vi "Dashboard Main.vi"() -> ()   [LabVIEW 2015]
uses:
  Camera Types.ctl
  <vilib>/Utility/miscctls.llb/LVRowAndColumnTypeDef.ctl
  <vilib>/event_ctls.llb/eventvkey.ctl
  <vilib>/Rock Robotics/WPI/Dashboard/WPI_DashboardLogging Global.vi
  <vilib>/Rock Robotics/Network Tables/NT Read Boolean.vi
  <vilib>/Utility/file.llb/Write Delimited Spreadsheet (DBL).vi
  <vilib>/Rock Robotics/Network Tables/NT Write Numeric Array.vi
  <vilib>/Utility/file.llb/Read Delimited Spreadsheet (DBL).vi
  <vilib>/Rock Robotics/Network Tables/NT Write Boolean.vi
  <vilib>/Utility/config.llb/Write Key (String).vi
  <vilib>/Utility/config.llb/Write Key (I32).vi
  <vilib>/Utility/config.llb/NI_LVConfig.lvlib
  <vilib>/vision/NI_Vision_Development_Module.lvlib
panel:
  in  "Dashboard Tab":T1(tab)=enum."Commands"
  in  "Left / Right":bool
  out "Compass":dbl(knob) scale=-180.0..180.0
  out "Aimed?":bool
  out "position":dbl
  out "defense":dbl
  out "Have ball?":bool
  in  "Camera Settings":T2={"Frame Rate"=30, "Compression"=30, "Size"=1} {"Frame Rate" scale=1.0..30.0; "Size" items=["640x480", "320x240", "160x120"]}
  out "Mode":T3(ring)=enum."Auto Disabled"
  in  "DB Camera Config":bool
  out "fps":dbl format="%#.1g"
  out "Mbps":dbl format="%#.1g"
  out "Mbps LED":bool
  in  "Auto Position":i32(slide)=1 scale=1.0..5.0
  in  "Auto Defense":T4(ring)=enum."Low Bar"
  out "Detected Targets":T5(array[cluster]) {"Normalized Rect"."Numeric 5" format="%#_2g"; "Normalized Rect"."Numeric 3" format="%#_2g"; "Normalized Rect"."Numeric 2" format="%#_2g"; "Normalized Rect"."Numeric" format="%#_2g"}
  out "Masked":T6(plugin-control)
  out "Background":bool
  out "Qualified Particles":i32
  out "Highest Avg Score":dbl format="%#_3g"
  in  "Std Devs for Calibration":cluster{"H":dbl, "S":dbl, "V":dbl}={"H"=4.0, "S"=6.0, "V"=6.0}
  in  "Rec Mode":enum32{"Stop", "Record", "Playback"}(radio)
  in  "camSwitch?":bool
  in  "LED Color":T7={"Hue"={110.52399131877658, 148.6727294921875}, "Sat"={34.78571428571429, 255.0}, "Val"={91.07142857142858, 255.0}} {"Hue" scale=0.0..255.0 scale format="%_1f"}
  in  "Annotate":bool=TRUE
  in  "Annotation Limit":dbl=75.0
  in  "Aspect Ratio Fudge Factor":dbl=1.0
  in  "Min Score Threshold":i32=70
  in  "Camera Type":T8=enum."1013"
  in  "Emphasize Limit Tests":bool=TRUE
  in  "Green BCG Values":T9={"Brightness"=128.0, "Contrast"=45.0, "Gamma"=1.0} {"Brightness" min=0 max=255 step=1 format="%.2f"; "Contrast" min=1 max=89 step=1 format="%.2f"; "Gamma" min=0.1 max=10 step=0.01 format="%.2f"}
  in  "Blue BCG Values":T9={"Brightness"=128.0, "Contrast"=45.0, "Gamma"=1.0} {"Brightness" min=0 max=255 step=1 format="%.2f"; "Contrast" min=1 max=89 step=1 format="%.2f"; "Gamma" min=0.1 max=10 step=0.01 format="%.2f"}
  in  "Red BCG Values":T9={"Brightness"=128.0, "Contrast"=45.0, "Gamma"=1.0} {"Brightness" min=0 max=255 step=1 format="%.2f"; "Contrast" min=1 max=89 step=1 format="%.2f"; "Gamma" min=0.1 max=10 step=0.01 format="%.2f"}
  in  "Vision":u16(ring) items=["Camera Off", "USB Camera SW", "USB Camera HW", "IP Camera"]
  in  "Save?":bool
  out "Tree":string(tree)
  in  "Test Slider":dbl(slide) scale=0.0..100.0 scale format="%#_3g"
  in  "On/Off":bool caption="Solenoid"
  in  "Test Name":u16(ring) items=["Select the test to run..."]
  in  "Test Tree":string(tree)
  in  "Motor":cluster{"Value":dbl, "Enable":bool} {"Value" scale=-1.0..1.0 scale format="%#_3g"}
  out "Progress":T10 {"Test Progress" scale=0.0..100.0}
  in  "Rev/Fwd":cluster{"Forward":bool, "Reverse":bool}
  in  "Test Ring":u16(ring) items=["Monochrome", "Color"]
  out "Cmd Status":string
  in  "Execute Command":bool
  in  "Command Params":string[][](table)
  in  "Command Selection":i32(listbox)
  out "NT Connection":bool
  in  "Select Auto":string(combo)
  in  "CheckList":i32(listbox)
  out "Original Image":T6(plugin-control)
  out "Camera Image":T6(plugin-control)
  in  "TCP":refnum<k5>
  out "Camera IP":string
  out "Image Message":string="Timeout in Camera Communications"
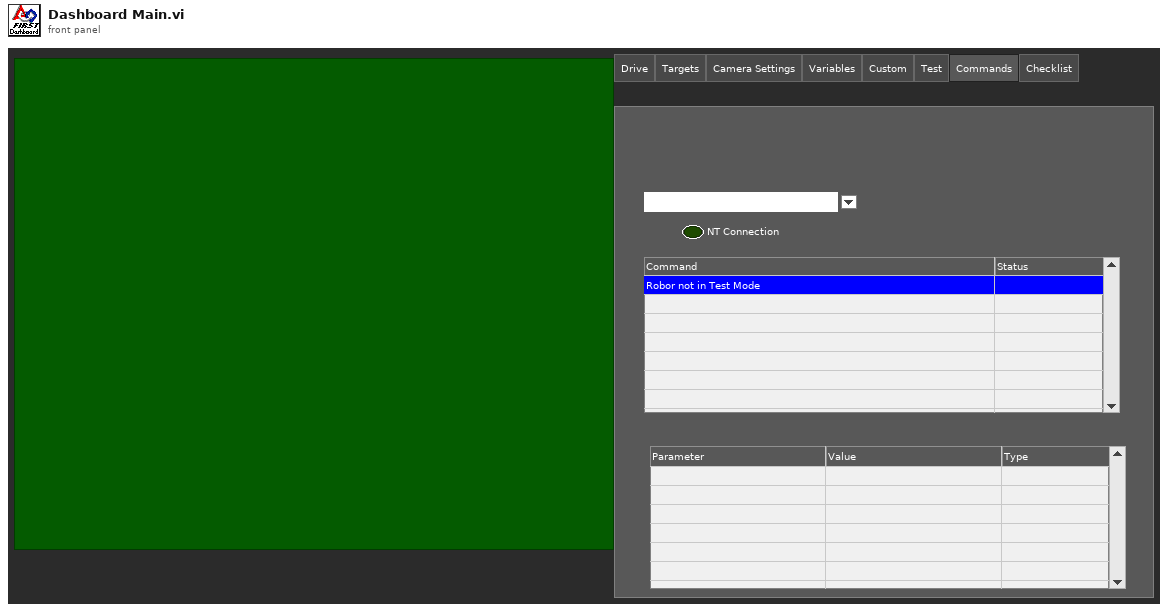
[diagram p1: front panel]
types:
  T1 = enum32{"Drive", "Targets", "Camera Settings", "Variables", "Custom", "Test", "Commands", "Checklist"}
  T2 = cluster{"Frame Rate":i32, "Compression":i32, "Size":u16}
  T3 = enum8{"Tele-Op Disabled", "Tele-Op Enabled", "Auto Disabled", "Auto Enabled", "Test Disabled", "Test Enabled", "Disconnected", "No Code", "E-Stop"}
  T4 = enum16{"Portcullis", "Cheval de Frise", "Low Bar", "Rock Wall", "Rough Terrain", "Moat", "Ramparts", "Vision Low Bar", "2-ball", "Do Nothing"}
  T5 = cluster{"Distance (ft)":dbl, "Center":cluster{dbl, dbl}, "Normalized Rect":cluster{"Numeric":dbl, "Numeric 2":dbl, "Numeric 3":dbl, "Numeric 5":dbl}}[]
  T6 = typedef "IMAQ Image.ctl" = refnum<image>
  T7 = cluster{"Hue":cluster{dbl, dbl}, "Sat":cluster{dbl, dbl}, "Val":cluster{dbl, dbl}}
  T8 = typedef "Camera Types.ctl" = enum16{"206", "1011", "1013", "MS HD3000 square", "MS HD3000 640x480"}
  T9 = cluster{"Brightness":sgl, "Contrast":sgl, "Gamma":sgl}
  T10 = cluster{"Test Progress":u8, "Test Progress Text":string}
  T11 = typedef "Image Type" = u32
  T12 = cluster{"IDs":cluster{"RPC field ID":u16, "Unique ID":u16}, "String":string}
  T13 = enum32{"Drive", "Basic", "Custom", "Test", "Checklist", "Variables"}
  T14 = cluster{cluster{"Numeric":dbl, "Numeric":dbl}, cluster{"Numeric":dbl, "Numeric":dbl}, cluster{"Numeric":dbl, "Numeric":dbl}}
  T15 = cluster{"Camera Image":refnum<vi>, "Dashboard Tab":refnum<vi>, "Background":refnum<vi>, "Vision":refnum<vi>, "Rec Mode":refnum<vi>, "Test Slider":refnum<vi>, "On/Off ":refnum<vi>, "Test Ring":refnum<vi>, "Rev/Fwd":refnum<vi>, "Test Name":refnum<vi>, "Motor":refnum<vi>, "Progress":refnum<vi>, "CheckList":refnum<vi>, "Tree":refnum<vi>, "Test Tree":refnum<vi>, "Command Params":refnum<vi>, "Command Selection":refnum<vi>, "Execute Command":refnum<vi>, "Cmd Status":refnum<vi>}
  T16 = typedef "Particle Parameters" = i32
  T17 = cluster{cluster{dbl, dbl}, cluster{dbl, dbl}, cluster{dbl, dbl}}
  T18 = cluster{"Bounding box":cluster{"left":dbl, "top":dbl, "right":dbl, "bottom":dbl}, "Aspect Ratio":dbl, "Area to CH":dbl, "X Mask":dbl, "Y Mask":dbl, "Moment":dbl}[]
  T19 = cluster{"Distance (ft)":dbl, "Center":cluster{dbl, dbl}, "Normalized Rect":cluster{"Numeric":dbl, "Numeric 2":dbl, "Numeric 3":dbl, "Numeric 5":dbl}}
  T20 = cluster{"Numeric":dbl, "Numeric 2":dbl, "Numeric 3":dbl, "Numeric 5":dbl}
  T21 = typedef "NI_LVConfig.lvlib/Config Data RefNum.ctl" = refnum<k1>
  T22 = cluster{"Error Strings":string, "Disable Counts":cluster{u16, u16}, "Rail Faults":cluster{u16, u16, u16}, "Robot IP":string, "DB Mode":u8, "Event Info":cluster{"Name":string, "Type":u8, "Number":u16, "Replay":u8}, "Camera Addr":string}
  T23 = cluster{"Storage":cluster{"Disk Free":u64, "RAM Block":u32, "RAM free":u32}, "CPU Utilization":cluster{"CPU % ISR":sgl, "CPU % Time Crit":sgl, "CPU % Timed Str":sgl, "CPU % High":sgl, "CPU % Above":sgl, "CPU % Normal":sgl, "CPU % Low":sgl}, "CAN":cluster{"% Bus Utilization":sgl, "Bus Off Cnt":u32, "TX_FIFO Full Cnt":u32, "Receive Error Cnt":u8, "Transmit Error Cnt":u8}, "HID":cluster{"HID Outputs":u32, "Rumble Low":u16, "Rumble High":u16}[]}
  T24 = cluster{"Status bits":cluster{"Test Mode":bool, "Autonomous":bool, "Enabled":bool, "Code Start":bool, "Brownout":bool, "Reserved 2":bool, "Reserved 3":bool, "E-Stop":bool}, "Code Trace":cluster{"Disabled":bool, "TeleOp":bool, "Auto":bool, "Test":bool}, "Controller Type":enum16{"unknown", "cRIO", "roboRio"}, "Code?":enum16{"unknown", "noCode", "code"}, "Battery V":dbl}
  T25 = cluster{"Control Bits":cluster{"TestMode":bool, "Autonomous":bool, "Enabled":bool, "FMS Present":bool, bool, bool, bool, "E-Stop":bool}, "Team Station ":u8, "Countdown":sgl, "Joystick Values":cluster{"Axes":dbl[], "Buttons":bool[], "POVs":i16[]}[]}
  T26 = cluster{"Operation":enum16{"Update", "Clear"}, "Color Box":u32}[]
  T27 = typedef "eventvkey.ctl" = enum16{"ASCII", "Enter", "Return", "Shift", "Ctrl", "Alt", "Cmd", "Opt", "Caps", "NumLock", "Clear", "Break", "Up", "Down", "Left", "Right", "Insert", "Delete", "Home", "End", "PageUp", "PageDown", "Escape", "Help", "Pause", "ScrollLock", "F1", "F2", "F3", "F4", "F5", "F6", "F7", "F8", "F9", "F10", "F11", "F12", "F13", "F14", "F15", "F16", "F17", "F18", "F19", "F20", "F21", "F22", "F23", "F24", "Play", "VolumeUp", "VolumeDown", "Mute", "Two Byte Char"}
  T28 = cluster{"Image Size":bool, "Image Type":bool, "Pixel Value":bool, "ROI Information":bool, "Zoom Factor":bool}
  T29 = enum8{"Enabled", "Disabled", "Disabled and Grayed Out"}
  T30 = cluster{"Operation":enum16{"Update", "Clear"}, "Color Box":u32}
  T31 = typedef "LVRowAndColumnTypeDef.ctl" = cluster{"Row":i32, "Column":i32}
  T32 = cluster{"Shift":bool, "Ctrl":bool, "Alt":bool, "Cmd":bool, "Opt":bool}
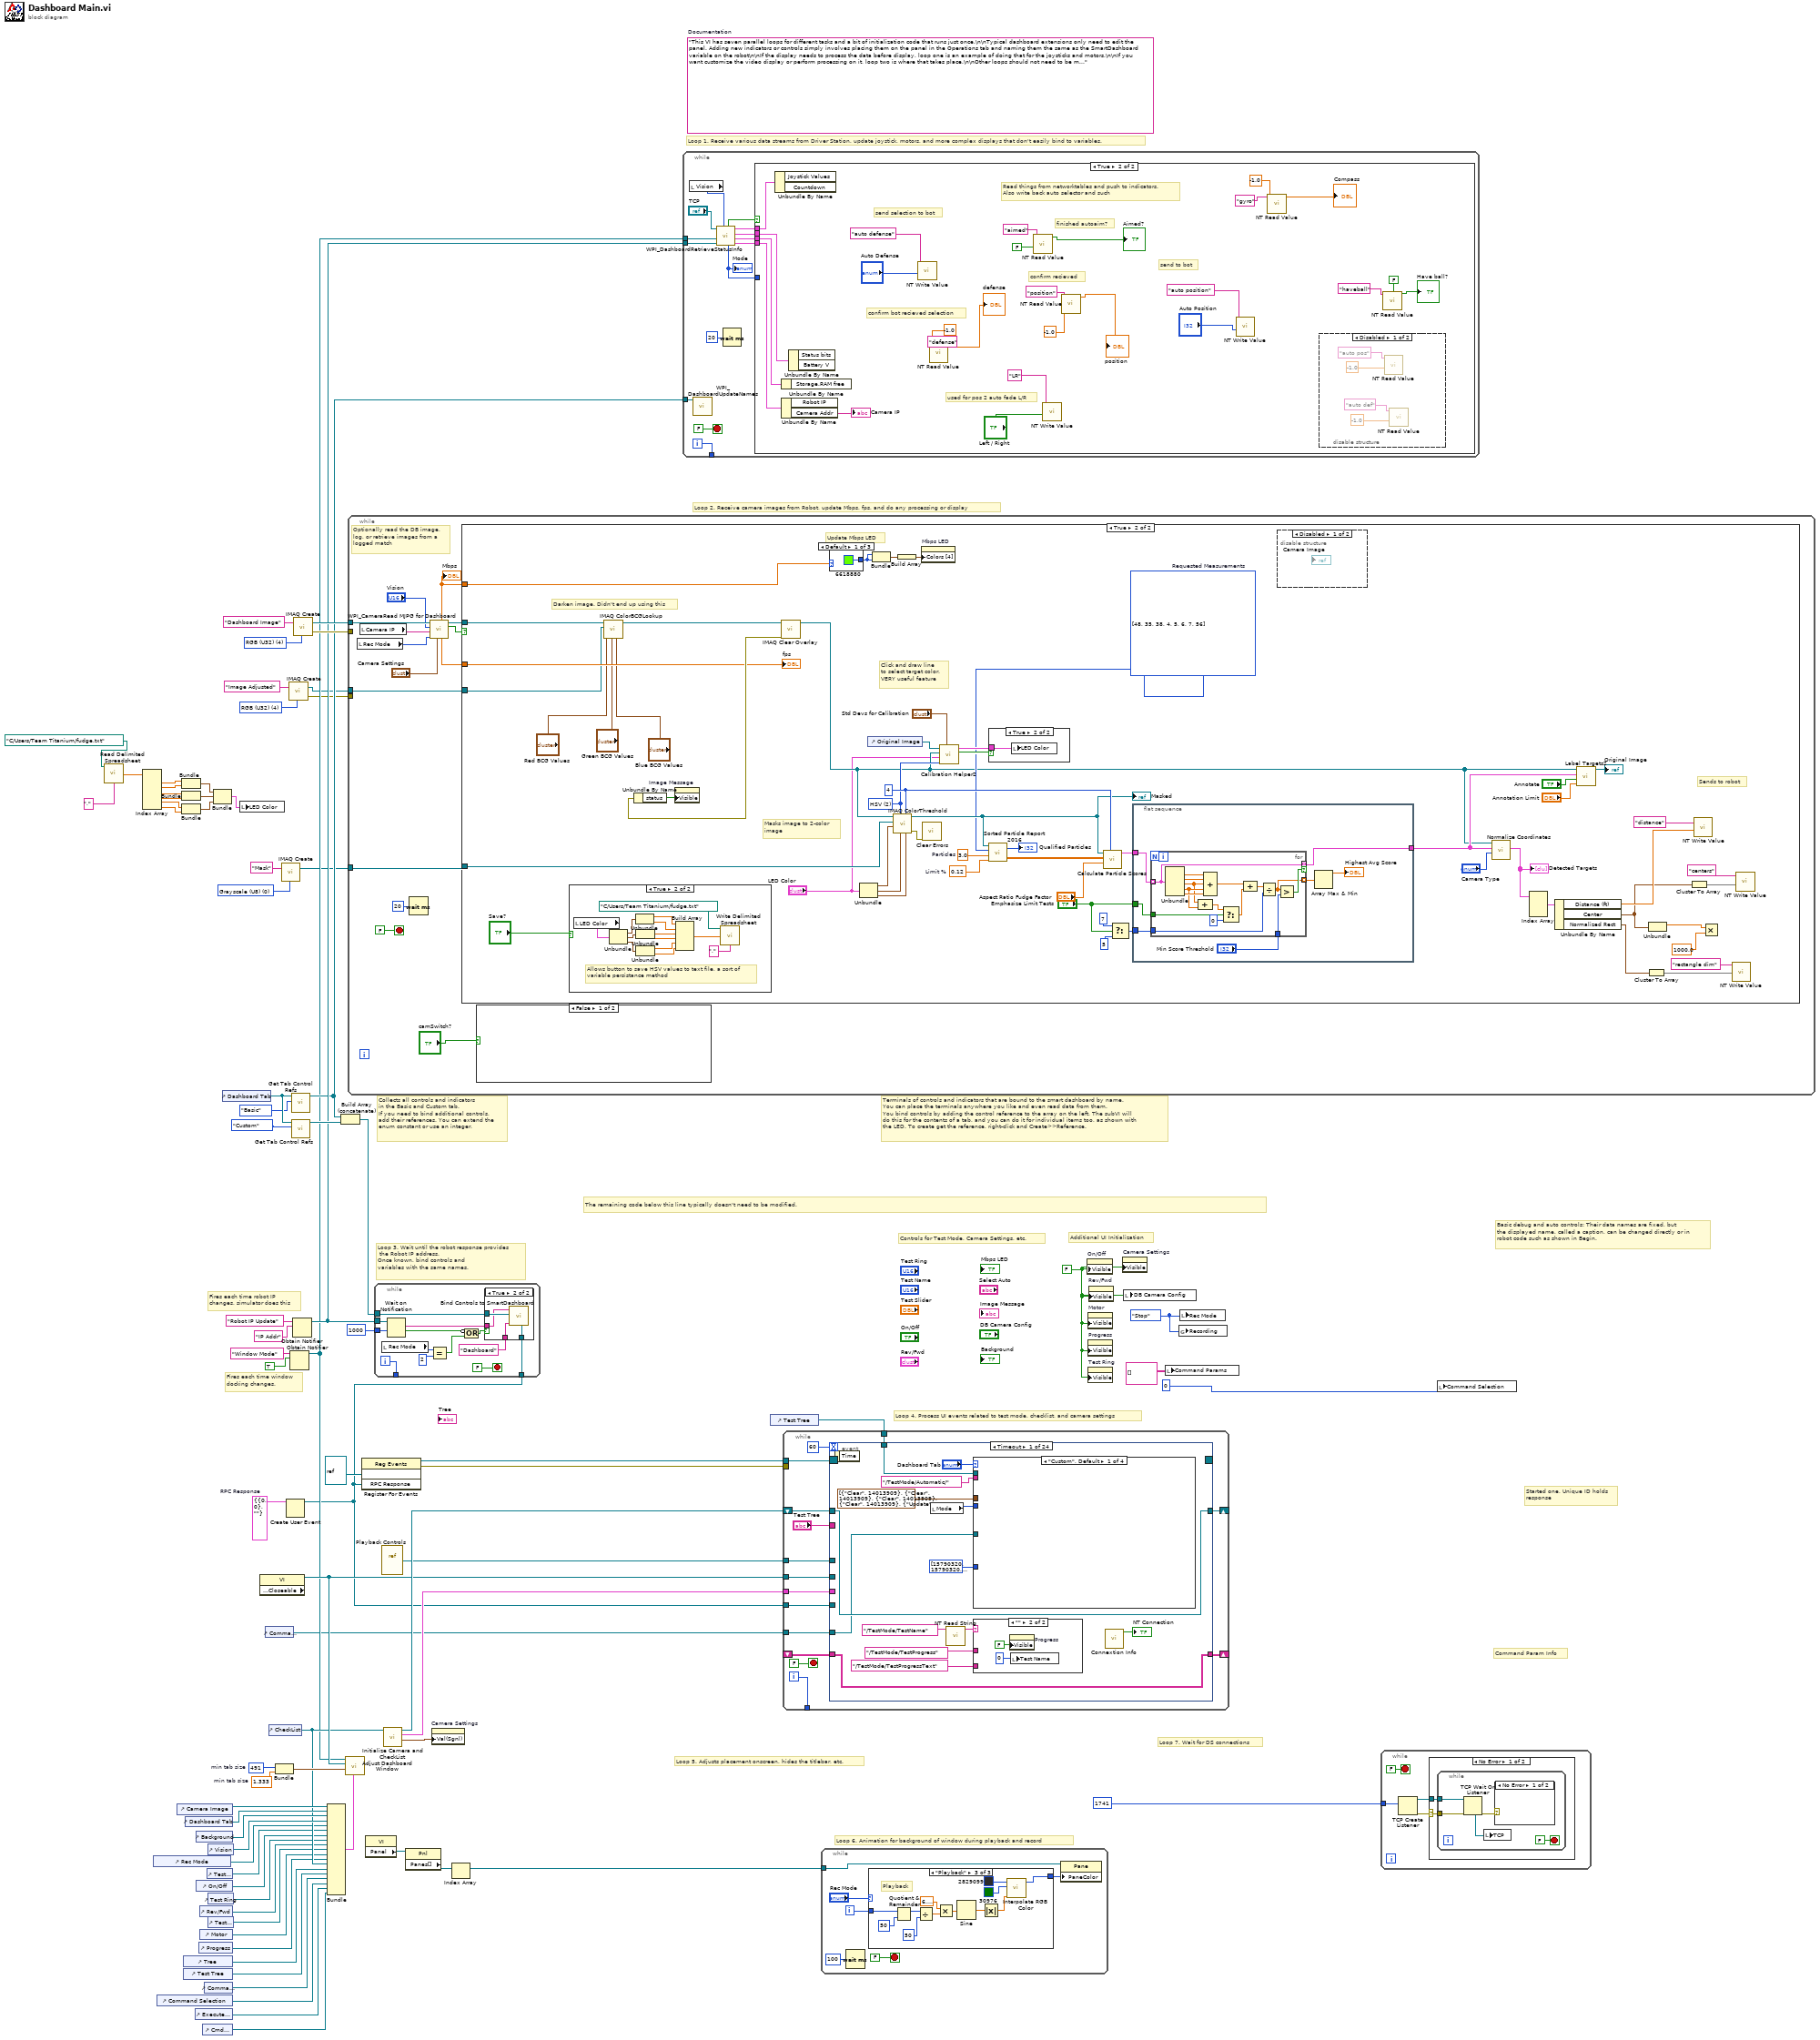
[diagram p0: block diagram]
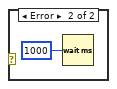
[diagram p2: hidden frame]
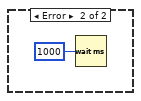
[diagram p3: hidden frame]
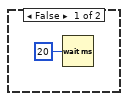
[diagram p4: hidden frame]
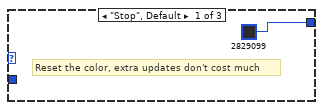
[diagram p6: hidden frame]
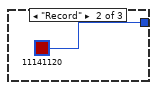
[diagram p7: hidden frame]
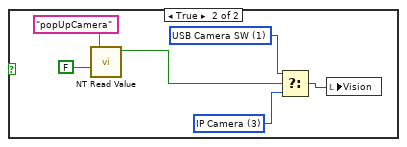
[diagram p9: hidden frame]
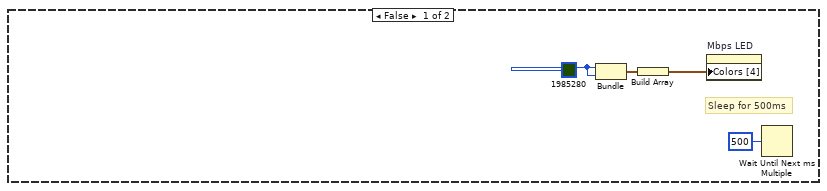
[diagram p10: hidden frame]
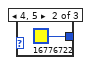
[diagram p14: hidden frame]
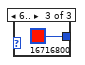
[diagram p15: hidden frame]
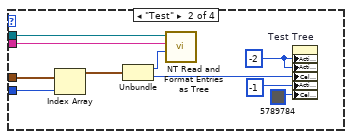
[diagram p16: hidden frame]
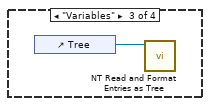
[diagram p17: hidden frame]
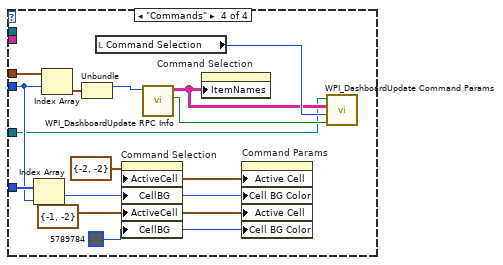
[diagram p18: hidden frame]
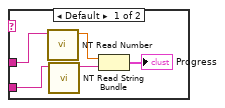
[diagram p19: hidden frame]
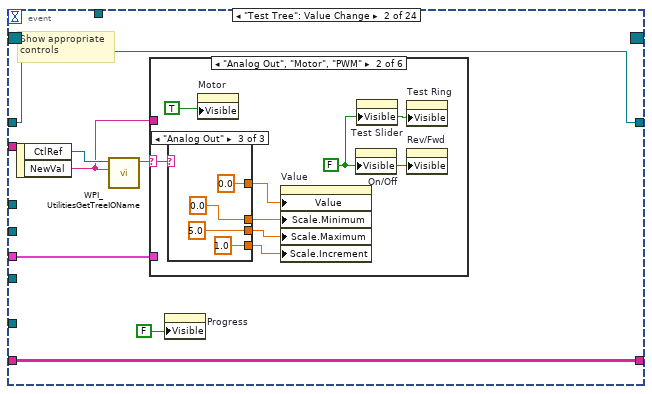
[diagram p20: hidden frame]
diagram:
  w17 = T11 4 items=["Grayscale (U8)", "Grayscale (I16)", "Grayscale (SGL)", "Complex (CSG)", "RGB (U32)", "HSL (U32)", "RGB (U64)"] ("Image Type")
  w19 = T11 0 items=["Grayscale (U8)", "Grayscale (I16)", "Grayscale (SGL)", "Complex (CSG)", "RGB (U32)", "HSL (U32)", "RGB (U64)", "Grayscale (U16)"] ("Image Type")
  w27 = T12 {"IDs"={"RPC field ID"=0, "Unique ID"=0}, "String"=""}  # RPC Response
  w52 = 491  # min tab size
  w51 = 1.333  # min tab size
  w60 = enum32{"Stop", "Record", "Playback"}."Stop" ("Rec Mode")
  w34 = FALSE ("Visible")
  (unwired) "This VI has seven parallel loops for different tasks and a bit of initialization code that runs just once.\n\nTypical dashboard extensions only need to edit the panel. Adding new indicators or controls simply involves placing them on the panel in the Operations tab and naming them the same as the SmartDashboard variable on the robot\n\nIf the display needs to process the data before display, loop one is an example of doing that for the joysticks and motors.\n\nIf you want customize the video display or perform processing on it, loop two is where that takes place.\n\nOther loops should not need to be modified. They are pretty standard, and document the task they perform."  # Documentation
  w80 = T11 4 items=["Grayscale (U8)", "Grayscale (I16)", "Grayscale (SGL)", "Complex (CSG)", "RGB (U32)", "HSL (U32)", "RGB (U64)"] ("Image Type")
  # "Command Param Info"
  # "Started one, Unique ID holds\nresponse"
  # "Loop 7. Wait for DS connections"
  # "Basic debug and auto controls: Their data names are fixed, but\nthe displayed name, called a caption, can be changed directly or in\nrobot code such as shown in Begin."
  # "Controls for Test Mode, Camera Settings, etc."
  # "Additional UI Initialization"
  # "Loop 6. Animation for background of window during playback and record"
  # "Fires each time robot IP\nchanges, simulator does this"
  # "Fires each time window\ndocking changes."
  # "Collects all controls and indicators\nin the Basic and Custom tab.\nIf you need to bind additional controls,\nadd their references. You can extend the\nenum constant or use an integer."
  # "The remaining code below this line typically doesn't need to be modified."
  # "Loop 4. Process UI events related to test mode, checklist, and camera settings"
  # "Terminals of controls and indicators that are bound to the smart dashboard by name.\nYou can place the terminals anywhere you like and even read data from them.\nYou bind controls by adding the control reference to the array on the left. The subVI will\ndo this for the contents of a tab, and you can do it for individual items too, as shown with\nthe LED. To create get the reference, right-click and Create>>Reference."
  # "Loop 3. Wait until the robot response provides\n the Robot IP address.\nOnce known, bind controls and\nvariables with the same names."
  # "Loop 5. Adjusts placement onscreen, hides the titlebar, etc."
  # "Loop 1. Receive various data streams from Driver Station, update joystick, motors, and more complex displays that don't easily bind to variables."
  # "Loop 2. Receive camera images from Robot, update Mbps, fps, and do any processing or display"
  n1 = call-poly <vilib>:"Read Delimited Spreadsheet.vi"("file path (dialog if empty)"=path "C:/Users/Team Titanium/fudge.txt", "delimiter (\\t)"="," ("delimiter (\\t)")) -> ("first row"=w12:dbl[])  [unwired: 8 in, 5 out]
  n2 = Index Array(array=w12) -> (element #1=w11:dbl, element #2=w10:dbl, element #3=w9:dbl, element #4=w8:dbl, element #5=w7:dbl, element #6=w6:dbl)  [unwired: 6 in]
  n3 = control-ref of="Rec Mode"() -> (w40:refnum<vi>)
  n4 = control-ref of="Command Selection"() -> (w26:refnum<vi>)
  n5 = control-ref of="Camera Image"() -> (w55:refnum<vi>)
  n6 = Bundle("Numeric"=w11, "Numeric"=w10) -> (w5:cluster{"Numeric":dbl, "Numeric":dbl})  [unwired: 1 in]
  n7 = Bundle("Numeric"=w9, "Numeric"=w8) -> (w4:cluster{"Numeric":dbl, "Numeric":dbl})  [unwired: 1 in]
  n8 = Bundle("Numeric"=w7, "Numeric"=w6) -> (w3:cluster{"Numeric":dbl, "Numeric":dbl})  [unwired: 1 in]
  n9 = control-ref of="Tree"() -> (w44:refnum<vi>)
  n10 = control-ref of="Test Tree"() -> (w43:refnum<vi>)
  n11 = control-ref of="Dashboard Tab"() -> (w54:refnum<vi>)
  n12 = control-ref of="Execute Command"() -> (w28:refnum<vi>)
  n13 = control-ref of="Background"() -> (w49:refnum<vi>)
  n14 = control-ref of="On/Off"() -> (w38:refnum<vi>)
  n15 = control-ref of="Progress"() -> (w35:refnum<vi>)
  n16 = control-ref of="Rev/Fwd"() -> (w36:refnum<vi>)
  n17 = control-ref of="Motor"() -> (w41:refnum<vi>)
  n18 = control-ref of="Cmd Status"() -> (w22:refnum<vi>)
  n19 = control-ref of="Command Params"() -> (w29:refnum<vi>)
  n20 = control-ref of="Test Slider"() -> (w39:refnum<vi>)
  n21 = control-ref of="Vision"() -> (w53:refnum<vi>)
  n22 = control-ref of="Test Ring"() -> (w37:refnum<vi>)
  n23 = control-ref of="Test Name"() -> (w42:refnum<vi>)
  n24 = Bundle(w5, w4, w3) -> (w2:T14)  [unwired: 1 in]
  n25 = control-ref of="Dashboard Tab"() -> (w58:refnum<vi>)
  n26 = local write "LED Color"(w2) -> ()
  n27 = property class="VI" props=["Front Panel.Closeable"]() -> (reference out=w59:refnum<vi>)  [unwired: 2 in, 2 out]
  n28 = control-ref of="Command Params"() -> (w21:refnum<vi>)
  n29 = control-ref of="CheckList"() -> (w45:refnum<vi>)
  n30 = Bundle("min tab size"=w52, "min tab size"=w51) -> (w50:cluster{"min tab size":i32, "min tab size":dbl})  [unwired: 1 in]
  n31 = call "IMAQ Create"("Image Name"="Mask", "Image Type"=w19) -> ("New Image"=w18:T6)  [unwired: 2 in, 2 out]
  n32 = Create User Event(user event datatype=w27) -> (user event=w23:refnum<user-event>)  [unwired: 1 in, 1 out]
  n33 = call "IMAQ Create"("Image Name"="Image Adjusted", "Image Type"=w17) -> ("New Image"=w15:T6, "error out"=w14:errorcluster)  [unwired: 2 in, 1 out]
  n34 = Obtain Notifier(name (unnamed)="Window Mode", notification data type=TRUE) -> (notifier out=w31:refnum<notifier>)  [unwired: 2 in, 2 out]
  n35 = call <vilib>:"Get Tab Control Refs.vi"("Page Index"=T13."Basic" ("Dashboard Tab"), "TabControl in"=w58) -> ("ControlsOnPage"=w32:refnum<vi>[])  [unwired: 9 in]
  n36 = call <vilib>:"Get Tab Control Refs.vi"("Page Index"=T13."Custom" ("Dashboard Tab"), "TabControl in"=w58) -> ("ControlsOnPage"=w57:refnum<vi>[])  [unwired: 9 in]
  n37 = Obtain Notifier(name (unnamed)="Robot IP Update", notification data type="IP Addr" ("name (unnamed)")) -> (notifier out=w33:refnum<notifier>)  [unwired: 2 in, 2 out]
  n38 = call "IMAQ Create"("Image Name"="Dashboard Image", "Image Type"=w80) -> ("New Image"=w78:T6, "error out"=w77:errorcluster)  [unwired: 2 in, 1 out]
  n39 = Bundle("Camera Image"=w55, "Dashboard Tab"=w54, "Background"=w49, "Vision"=w53, "Rec Mode"=w40, "Test Slider"=w39, "On/Off"=w38, "Test Ring"=w37, "Rev/Fwd"=w36, "Test Name"=w42, "Motor"=w41, "Progress"=w35, "CheckList"=w45, "Tree"=w44, "Test Tree"=w43, "Command Params"=w29, "Command Selection"=w26, "Execute Command"=w28, "Cmd Status"=w22) -> (w46:T15)  [unwired: 1 in]
  n40 = Build Array (concatenate)(w32, w57) -> (w56:refnum<vi>[])
  n41 = call "Adjust Dashboard Window.vi"("Sizing Refnums"=w46, "Size Constraints"=w50, "VI"=w59, "WIn Mode"=w31) -> ()  [unwired: 8 in]
  n42 = while {
    tunnel: w78 -> [w94]
    tunnel: w77 -> [_]
    tunnel: w18 -> [w84]
    tunnel: w15 -> [w83]
    tunnel: w14 -> [_]
    stop <- FALSE stop-if-true
    # "Optionally read the DB image,\nlog, or retrieve images from a\nlogged match"
    n43 = local read "Rec Mode"() -> (w89:enum32{"Stop", "Record", "Playback"})
    n44 = local read "Camera IP"() -> (w87:string)
    n45 = Wait (ms)(milliseconds to wait=u32 20) -> ()  [unwired: 1 out]
    n46 = call <vilib>:"WPI_CameraRead MJPG for Dashboard.vi"("Camera Settings"="Camera Settings", "Rec Mode"=w89, "Camera IP"=w87, "Camera Mode"="Vision", "Refnum in"=w94) -> ("Active"=w92:bool, "Refnum out"=w93:T6, "FPS"=w91:dbl, "Bandwidth (Mbps)"=w86:dbl)  [unwired: 3 in]
    "Mbps" <- w86
    n47 = case shown="True" w92 {
      tunnel: w93 -> [_ w124]
      tunnel: w86 -> [_ w155]
      tunnel: w91 -> [_ w154]
      tunnel: w84 -> [_ w128]
      tunnel: w83 -> [_ w122]
      frame False {
        w101 = u32 1985280 ("Color Box")
        # "Sleep for 500ms"
        n48 = Bundle("Color Box"=w101, "Color Box"=w101) -> (w103:cluster{"Color Box":u32, "Color Box":u32})  [unwired: 1 out]
        n49 = Build Array(w103) -> (w102:cluster{"Color Box":u32, "Color Box":u32}[])
        n50 = property on="Mbps LED" class="Bool (strict)"("Colors [4]"=w102) -> ()  [unwired: 2 in, 2 out]
        n51 = Wait Until Next ms Multiple(millisecond multiple=u32 500) -> ()  [unwired: 1 out]
      }
      frame True {
        w127 = T16[] [48, 35, 38, 4, 5, 6, 7, 56] items=["Center of Mass X", "Center of Mass Y", "First Pixel X", "First Pixel Y", "Bounding Rect Left", "Bounding Rect Top", "Bounding Rect Right", "Bounding Rect Bottom", "Max Feret Diameter Start X", "Max Feret Diameter Start Y", "Max Feret Diameter End X", "Max Feret Diameter End Y", "Max Horiz. Segment Length Left", "Max Horiz. Segment Length Right", "Max Horiz. Segment Length Row", "-", "Bounding Rect Width", "Bounding Rect Height", "Bounding Rect Diagonal", "Perimeter", "Convex Hull Perimeter", "Holes' Perimeter", "Max Feret Diameter", "Equivalent Ellipse Major Axis", "Equivalent Ellipse Minor Axis", "Equivalent Ellipse Minor Axis (Feret)", "Equivalent Rect Long Side", "Equivalent Rect Short Side", "Equivalent Rect Diagonal", "Equivalent Rect Short Side (Feret)", "Average Horiz. Segment Length", "Average Vert. Segment Length", "Hydraulic Radius", "Waddel Disk Diameter", "-", "Area", "Holes' Area", "Particle & Holes' Area", "Convex Hull Area", "Image Area", "-", "Number of Holes", "Number of Horiz. Segments", "Number of Vert. Segments", "-", "Orientation", "Max Feret Diameter Orientation", "-", "% Area/Image Area", "% Area/(Particle & Holes' Area)", "Ratio of Equivalent Ellipse Axes", "Ratio of Equivalent Rect Sides", "-", "Elongation Factor", "Compactness Factor", "Heywood Circularity Factor", "Type Factor", "-", "Sum X", "Sum Y", "Sum XX", "Sum XY", "Sum YY", "Sum XXX", "Sum XXY", "Sum XYY", "Sum YYY", "-", "Moment of Inertia XX", "Moment of Inertia XY", "Moment of Inertia YY", "Moment of Inertia XXX", "Moment of Inertia XXY", "Moment of Inertia XYY", "Moment of Inertia YYY", "Norm. Moment of Inertia XX", "Norm. Moment of Inertia XY", "Norm. Moment of Inertia YY", "Norm. Moment of Inertia XXX", "Norm. Moment of Inertia XXY", "Norm. Moment of Inertia XYY", "Norm. Moment of Inertia YYY", "Hu Moment 1", "Hu Moment 2", "Hu Moment 3", "Hu Moment 4", "Hu Moment 5", "Hu Moment 6", "Hu Moment 7"]  # Requested Measurements
        w145 = 4 ("Replace Value")
        w147 = 0.12  # Limit %
        w150 = 3.0  # Particles
        w131 = u16 2 items=["RGB", "HSL", "HSV", "HSI"] ("Color Mode")
        # "Sends to robot"
        # "Masks image to 2-color\nimage"
        # "Darken image. Didn't end up using this"
        # "Click and draw line\nto select target color.\nVERY useful feature"
        # "Update Mbps LED"
        n52 = case shown="True" "Save?" {
          frame False {
          }
          frame True {
            # "Allows button to save HSV values to text file, a sort of\nvariable persistance method"
            n53 = local read "LED Color"() -> (w161:T7)
            n54 = Unbundle(w161) -> ("Hue"=w167:cluster{dbl, dbl}, "Sat"=w166:cluster{dbl, dbl}, "Val"=w165:cluster{dbl, dbl})
            n55 = Unbundle(w167) -> (w173:dbl, w172:dbl)
            n56 = Unbundle(w166) -> (w171:dbl, w170:dbl)
            n57 = Unbundle(w165) -> (w169:dbl, w168:dbl)
            n58 = Build Array(w173, w172, w171, w170, w169, w168) -> (w163:dbl[])
            n59 = call-poly <vilib>:"Write Delimited Spreadsheet.vi"("file path (dialog if empty)"=path "C:/Users/Team Titanium/fudge.txt", "1D data"=w163, "delimiter (\\t)"="," ("delimiter (\\t)")) -> ()  [unwired: 11 in, 2 out]
          }
        }
        n60 = call "IMAQ ColorBCGLookup"("Blue BCG Values"="Blue BCG Values", "Green BCG Values"="Green BCG Values", "Red BCG Values"="Red BCG Values", "Image Dst"=w122, "Image Src"=w124) -> ("Image Dst Out"=w123:T6)  [unwired: 5 in, 1 out]
        n61 = call "IMAQ Clear Overlay"("Image"=w123) -> ("error out"=w159:errorcluster, "Image Out"=w125:T6)  [unwired: 2 in, 7 out]
        n62 = Unbundle By Name(w159) -> ("status"=w160:bool)
        n63 = property on="Image Message" class="Str"("Visible"=w160) -> ()  [unwired: 2 in, 2 out]
        n64 = case shown="Default" w155 {
          tunnel: [u32 6618880 ("Color Box") u32 16776722 ("Color Box") u32 16716800 ("Color Box")] -> w156
          frame Default {
          }
          frame 4, 5 {
          }
          frame 6.. {
          }
        }
        n65 = Unbundle("LED Color") -> ("Hue"=w153:cluster{dbl, dbl}, "Sat"=w152:cluster{dbl, dbl}, "Val"=w151:cluster{dbl, dbl})
        n66 = control-ref of="Original Image"() -> (w134:refnum<vi>)
        n67 = Bundle("Color Box"=w156, "Color Box"=w156) -> (w158:cluster{"Color Box":u32, "Color Box":u32})  [unwired: 1 out]
        n68 = call "IMAQ ColorThreshold"("Blue or Luma or Val or Inten Range"=w151, "Replace Value"=w145, "Green or Sat Range"=w152, "Color Mode"=w131, "Red or Hue Range"=w153, "Image Dst"=w128, "Image Src"=w125) -> ("error out"=w138:errorcluster, "Image Dst Out"=w139:T6)  [unwired: 3 in]
        "Masked" <- w139
        n69 = Build Array(w158) -> (w157:cluster{"Color Box":u32, "Color Box":u32}[])
        n70 = property on="Mbps LED" class="Bool (strict)"("Colors [4]"=w157) -> ()  [unwired: 2 in, 2 out]
        n71 = call <vilib>:"Clear Errors.vi"("error in (no error)"=w138) -> ()  [unwired: 5 in, 2 out]
        n72 = call "Calibration Helper2.vi"("Std Devs"="Std Devs for Calibration", "Color Mode"=w131, "Color Components"="LED Color", "Image"=w125, "Image Ctl Refnum"=w134) -> ("Changed"=w133:bool, "output color"=w132:T17)  [unwired: 5 in]
        n73 = call "Sorted Particle Report 2016.vi"("Min Area Size %"=w147, "Particle Count Limit"=w150, "Pixel Measurements"=w127, "Image in"=w139) -> ("Sorted Data"=w148:dbl[][], "Particles"=→"Qualified Particles":i32)
        n74 = case shown="True" w133 {
          tunnel: w132 -> [_ w174]
          frame False {
          }
          frame True {
            n75 = local write "LED Color"(w174) -> ()
          }
        }
        n76 = call "Calculate Particle Scores.vi"("Pixel Value"=w145, "Aspect Fudge Factor"="Aspect Ratio Fudge Factor", "Sorted Data"=w148, "Image in"=w139) -> ("Scores"=w142:T18)  [unwired: 7 in]
        n77 = Select(t=7, s="Emphasize Limit Tests", f=5) -> (s? t:f=w135:i32)
        n78 = flat-sequence {
          tunnel: w142 -> [w180]
          tunnel: [w181] -> w140
          tunnel: w135 -> [w177]
          tunnel: "Emphasize Limit Tests" -> [w175]
          frame #0 {
            n79 = for {
              tunnel: w180 -> [w195] mode=indexing
              tunnel: [w195] -> w181 mode=indexing if=w194
              tunnel: [w193] -> w179 mode=indexing
              tunnel: w177 -> [w192]
              tunnel: "Min Score Threshold" -> [w191]
              tunnel: w175 -> [w184]
              n80 = Unbundle(w195) -> ("Aspect Ratio"=w197:dbl, "Area to CH"=w196:dbl, "X Mask"=w186:dbl, "Y Mask"=w187:dbl, "Moment"=w188:dbl)  [unwired: 1 out]
              n81 = Compound Arithmetic op=ADD(w186, w187) -> (w185:dbl)
              n82 = Compound Arithmetic op=ADD(w197, w196, w186, w187, w188) -> (w190:dbl)
              n83 = Select(t=w185, s=w184, f=0) -> (s? t:f=w183:dbl)
              n84 = Compound Arithmetic op=ADD(w190, w183) -> (w189:dbl)
              n85 = Divide(x=w189, y=w192) -> (x/y=w193:dbl)
              n86 = Greater?(x=w193, y=w191) -> (0:w194:bool)
            }
            n87 = Array Max & Min(array=w179) -> (max value=→"Highest Avg Score":dbl)  [unwired: 3 out]
          }
        }
        n88 = disable-structure shown="Disabled" {
          frame Disabled {
          }
          frame Enabled {
          }
        }
        n89 = call "Normalize Coordinates.vi"("Camera Type"="Camera Type", "Targets"=w140, "Image in"=w125) -> ("Found Targets"=w118:T5)  [unwired: 7 in, 1 out]
        "Detected Targets" <- w118
        n90 = Index Array(array=w118) -> (element #1=w117:T19)  [unwired: 3 in, 2 out]
        n91 = Unbundle By Name(w117) -> ("Distance (ft)"=w115:dbl, "Center"=w109:cluster{dbl, dbl}, "Normalized Rect"=w111:T20)
        n92 = call "Label Targets2.vi"("Score Threshold"="Annotation Limit", "Annotate"="Annotate", "Targets"=w140, "Image in"=w125) -> ("Image out"=→"Original Image":T6)  [unwired: 7 in]
        n93 = Cluster To Array(cluster=w111) -> (array=w110:dbl[])
        n94 = Unbundle(w109) -> (w107:dbl)  [unwired: 1 out]
        n95 = Cluster To Array(cluster=w109) -> (array=w113:dbl[])
        n96 = call-poly <vilib>:"NT Write Value.vi"("Numeric"=w115, "Name"="distance") -> ()  [unwired: 9 in, 1 out]
        n97 = Multiply(x=w107, y=1000.0) -> ()  [unwired: 1 out]
        n98 = call-poly <vilib>:"NT Write Value.vi"("Numeric Array"=w110, "Name"="rectangle dim") -> ()  [unwired: 9 in, 1 out]
        n99 = call-poly <vilib>:"NT Write Value.vi"("Numeric Array"=w113, "Name"="centers") -> ()  [unwired: 9 in, 1 out]
        "fps" <- w154
      }
    }
    n100 = case shown="False" "camSwitch?" {
      frame False {
      }
      frame True {
        w99 = u16 3 items=["Camera Off", "USB Camera SW", "USB Camera HW", "IP Camera"] ("Vision")
        w98 = u16 1 items=["Camera Off", "USB Camera SW", "USB Camera HW", "IP Camera"] ("Vision")
        n101 = call-poly <vilib>:"NT Read Value.vi"("Default Value"=FALSE, "Name"="popUpCamera") -> ("Boolean"=w100:bool)  [unwired: 8 in, 1 out]
        n102 = Select(t=w98, s=w100, f=w99) -> (s? t:f=w97:u16)
        n103 = local write "Vision"(w97) -> ()
      }
    }
  }
  n104 = register-events(refnum<vi> refnum, w23) -> (reference out=w64:refnum<event-registration>, error out=w63:errorcluster)  [unwired: 2 in]
  n105 = property class="VI"() -> ("Panel"=w67:refnum<vi>)  [unwired: 2 in, 2 out]
  n106 = while {
    tunnel: w56 -> [w213]
    tunnel: w33 -> [w211]
    tunnel: [w209] -> _
    tunnel: u32 1000 ("milliseconds to wait") -> [w208]
    tunnel: w23 -> [w201]
    i -> [w209]
    stop <- FALSE stop-if-true
    n107 = local read "Rec Mode"() -> (w204:enum32{"Stop", "Record", "Playback"})
    n108 = Wait on Notification(notifier=w211, timeout in ms (-1)=w208) -> (notification=w210:string, timed out?=w206:bool)  [unwired: 2 in, 2 out]
    n109 = Equal?(x=w204, y=u16 2 ("Rec Mode")) -> (x = y?=w205:bool)
    n110 = Compound Arithmetic op=OR(invert w206, w205) -> (w207:bool)
    n111 = case shown="True" w207 {
      tunnel: w213 -> [_ w217]
      tunnel: w210 -> [_ w216]
      tunnel: "Dashboard" -> [_ w215]
      tunnel: w201 -> [_ w214]
      frame False {
      }
      frame True {
        n112 = call <vilib>:"Bind Controls to SmartDashboard.vi"("RPC ref"=w214, "Client Name"=w215, "Bound Control Refs"=w217, "Server IP Address"=w216) -> ()  [unwired: 8 in]
      }
    }
  }
  n113 = vi-ref "Playback Controls.vi"() -> (w65:refnum<vi>)
  n114 = call "Initialize Camera and CheckList.vi"("ListBox in"=w45) -> ("Cluster"=w71:cluster{"value":i32, "value":i32, "index":i32}, "Array"=w72:cluster{string[]}[], "File Refnum"=w70:T21)  [unwired: 8 in]
  n115 = property class="Pnl"(reference=w67) -> ("Panes[]"=w68:refnum<vi>[])  [unwired: 1 in, 2 out]
  n116 = property on="Camera Settings" class="Clust (strict)"("Val(Sgnl)"=w71) -> ()  [unwired: 2 in, 2 out]
  n117 = Index Array(array=w68) -> (element=w66:refnum<vi>)  [unwired: 1 in]
  n118 = while {
    tunnel: [w230] -> _
    tunnel: w33 -> [w224]
    tunnel: w32 -> [w223]
    tunnel: w31 -> [w219]
    i -> [w230]
    stop <- FALSE stop-if-true
    n119 = local read "Vision"() -> (w221:u16)
    n120 = call <vilib>:"WPI_DashboardUpdateNames.vi"("Controls on Tab"=w223) -> ()  [unwired: 11 in]
    n121 = call <vilib>:"WPI_DashboardRetrieveStatusInfo.vi"("Vision"=w221, "Binding Refnum"=w224, "Window Mode Notifier"=w219, "TCP Cnx"="TCP") -> ("Power and Errors"=w225:T22, "Robot Metrics"=w228:T23, "Status Info"=w229:T24, "Control Info"=w226:T25, "Robot Mode"=w222:T3, "Process?"=w227:bool)  [unwired: 2 in]
    "Mode" <- w222
    n122 = Wait (ms)(milliseconds to wait=u32 20) -> ()  [unwired: 1 out]
    n123 = case shown="True" w227 {
      tunnel: w229 -> [_ w258]
      tunnel: w228 -> [_ w257]
      tunnel: w226 -> [_ w256]
      tunnel: w225 -> [_ w255]
      tunnel: w222 -> [_ _]
      frame False {
        n124 = Wait (ms)(milliseconds to wait=u32 20) -> ()  [unwired: 1 out]
      }
      frame True {
        # "used for pos 2 auto fade L/R"
        # "confirm recieved"
        # "send to bot"
        # "confirm bot recieved selection"
        # "send selection to bot"
        # "finished autoaim?"
        # "Read things from networktables and push to indicators.\nAlso write back auto selector and such"
        n125 = Unbundle By Name(w256) -> ()  [unwired: 2 out]
        n126 = Unbundle By Name(w257) -> ()  [unwired: 1 out]
        n127 = Unbundle By Name(w255) -> ("Camera Addr"=→"Camera IP":string)  [unwired: 1 out]
        n128 = Unbundle By Name(w258) -> ()  [unwired: 2 out]
        n129 = call-poly <vilib>:"NT Write Value.vi"("Numeric"="Auto Defense", "Name"="auto defense") -> ()  [unwired: 9 in, 1 out]
        n130 = call-poly <vilib>:"NT Read Value.vi"("Default Value"=-1.0, "Name"="defense") -> ("Numeric"=→"defense":dbl)  [unwired: 8 in, 1 out]
        n131 = call-poly <vilib>:"NT Read Value.vi"("Default Value"=FALSE, "Name"="aimed") -> ("Boolean"=→"Aimed?":bool)  [unwired: 8 in, 1 out]
        n132 = call-poly <vilib>:"NT Write Value.vi"("Boolean"="Left / Right", "Name"="LR") -> ()  [unwired: 9 in, 1 out]
        n133 = call-poly <vilib>:"NT Read Value.vi"("Default Value"=-1.0, "Name"="position") -> ("Numeric"=→"position":dbl)  [unwired: 8 in, 1 out]
        n134 = call-poly <vilib>:"NT Write Value.vi"("Numeric"="Auto Position", "Name"="auto position") -> ()  [unwired: 9 in, 1 out]
        n135 = call-poly <vilib>:"NT Read Value.vi"("Default Value"=-1.0, "Name"="gyro") -> ("Numeric"=→"Compass":dbl)  [unwired: 8 in, 1 out]
        n136 = disable-structure shown="Disabled" {
          frame Disabled {
            n137 = call-poly <vilib>:"NT Read Value.vi"("Default Value"=-1.0, "Name"="auto pos") -> ()  [unwired: 8 in, 2 out]
            n138 = call-poly <vilib>:"NT Read Value.vi"("Default Value"=-1.0, "Name"="auto def") -> ()  [unwired: 8 in, 2 out]
          }
          frame Enabled {
          }
        }
        n139 = call-poly <vilib>:"NT Read Value.vi"("Default Value"=FALSE, "Name"="haveball") -> ("Boolean"=→"Have ball?":bool)  [unwired: 8 in, 1 out]
      }
    }
  }
  n140 = control-ref of="Test Tree"() -> (w69:refnum<vi>)
  n141 = while {
    tunnel: w72 -> [w274]
    shift-right: [w273] -> _
    shift-left: w70 -> [w272]
    tunnel: [w271] -> _
    tunnel: w69 -> [w270]
    tunnel: w65 -> [w269]
    tunnel: w64 -> [w268]
    tunnel: w63 -> [_]
    tunnel: w59 -> [w267]
    tunnel: w23 -> [w266]
    tunnel: w21 -> [w265]
    shift-right: [w264] -> _
    shift-left: _ -> [w263]
    i -> [w271]
    stop <- FALSE stop-if-true
    n142 = event shown="[0] Timeout" {
      selector: w268 -> [_ _ _ _ _ _ _ _ _ _ _ _ _ _ _ _ _ _ _ _ _ _ _ _]
      dyn-events: [_ _ _ _ _ _ _ _ _ _ _ _ _ _ _ _ _ _ w583 _ _ _ _ _] -> _
      timeout: u32 60 ("milliseconds to wait") -> [_ _ _ _ _ _ _ _ _ _ _ _ _ _ _ _ _ _ _ _ _ _ _ _]
      tunnel: w270 -> [w287 _ _ _ _ _ _ _ _ _ _ _ _ _ _ _ _ _ _ _ _ _ _ _]
      tunnel: "Test Tree" -> [_ _ _ _ _ _ _ _ _ _ _ _ _ w546 w555 w558 w563 w572 _ _ _ _ _ _]
      tunnel: w274 -> [_ w325 _ _ _ _ _ _ _ _ _ w508 w539 _ _ _ _ _ _ _ _ _ _ _]
      tunnel: [w284 w324 w428 w434 w444 w448 w454 w466 w474 w480 w493 w507 w532 w545 w553 w557 w562 w571 w585 w601 w603 w611 w622 w627] -> w273
      tunnel: w272 -> [w284 w324 w428 w434 w444 w448 w454 w466 w474 w480 w493 w506 w532 w545 w553 w557 w562 w571 w585 w601 w603 w611 w622 w627]
      tunnel: w269 -> [_ _ _ _ _ _ _ _ _ _ _ _ _ _ _ _ _ _ w586 _ w606 _ _ _]
      tunnel: w267 -> [_ _ _ _ _ _ _ _ _ _ _ _ _ _ _ _ _ _ w581 _ _ _ _ _]
      tunnel: w266 -> [_ _ _ _ _ _ _ _ _ _ _ _ _ _ _ _ _ _ w577 _ _ _ _ _]
      tunnel: w265 -> [w279 _ _ _ _ _ w452 _ _ _ _ _ _ _ _ _ _ _ _ _ _ _ _ _]
      tunnel: [w278 w323 w427 w433 w443 w449 w450 w460 w471 w479 w492 w505 w531 w544 w552 w556 w561 w570 w576 w599 w602 w607 w615 w628] -> w264
      tunnel: w263 -> [w278 w323 w427 w433 w443 w449 w450 _ _ w479 w492 w505 w531 w544 w552 w556 w561 w570 w576 w599 w602 w607 w615 w628]
      event Timeout {
        n143 = event-data() -> ()  [unwired: 1 in, 1 out]
        n144 = local read "Mode"() -> (w281:T3)
        n145 = call <vilib>:"NT Read String.vi"("Name"="/TestMode/TestName") -> ("String"=w290:string)  [unwired: 9 in, 1 out]
        n146 = case shown="\"Custom\", Default" "Dashboard Tab" {
          tunnel: w287 -> [_ w301 _ _]
          tunnel: "/TestMode/Automatic/" ("Name Pattern") -> [_ w300 _ _]
          tunnel: T26 [{"Operation"=enum."Clear", "Color Box"=14013909}, {"Operation"=enum."Clear", "Color Box"=14013909}, {"Operation"=enum."Clear", "Color Box"=14013909}, {"Operation"=enum."Clear", "Color Box"=14013909}, {"Operation"=enum."Update", "Color Box"=14013909}, {"Operation"=enum."Update", "Color Box"=16777215}, {"Operation"=enum."Clear", "Color Box"=14013909}, {"Operation"=enum."Clear", "Color Box"=14013909}, {"Operation"=enum."Clear", "Color Box"=14013909}] -> [_ w293 _ w310]
          tunnel: w281 -> [_ w292 _ w309]
          tunnel: u32[] [15790320, 15790320, 15790320, 15790320, 16777215, 16777215, 15790320, 15790320, 15790320] -> [_ _ _ w315]
          tunnel: w279 -> [_ _ _ w303]
          frame "Custom", Default {
          }
          frame "Test" {
            w299 = -2 ("Active Item:Row Number")
            n147 = Index Array(array=w293, index=w292) -> (element=w294:T30)
            n148 = Unbundle(w294) -> ("Operation"=w295:enum16{"Update", "Clear"}, "Color Box"=w296:u32)
            n149 = call <vilib>:"NT Read and Format Entries as Tree.vi"("Operation"=w295, "Name Pattern"=w300, "Tree Refnum"=w301) -> ()  [unwired: 7 in, 2 out]
            n150 = property on="Test Tree" class="Tree (strict)"("Active Item Row Number"=w299, "ActiveColNum"=w299, "CellBG"=w296, "Active Item Row Number"=-1 ("Active Item:Row Number"), "CellBG"=u32 5789784 ("Color Box")) -> ()  [unwired: 2 in, 2 out]
          }
          frame "Variables" {
            n151 = control-ref of="Tree"() -> (w302:refnum<vi>)
            n152 = call <vilib>:"NT Read and Format Entries as Tree.vi"("Tree Refnum"=w302) -> ()  [unwired: 9 in, 2 out]
          }
          frame "Commands" {
            w311 = u32 5789784 ("Color Box")
            w312 = T31 {"Row"=-1, "Column"=-2} ("Active Cell:Active Cell")
            w314 = T31 {"Row"=-2, "Column"=-2} ("Active Cell:Active Cell")
            n153 = Index Array(array=w315, index=w309) -> (element=w313:u32)
            n154 = Index Array(array=w310, index=w309) -> (element=w308:T30)
            n155 = Unbundle(w308) -> ("Operation"=w307:enum16{"Update", "Clear"})  [unwired: 1 out]
            n156 = local read "Command Selection"() -> (w306:i32)
            n157 = property on="Command Selection" class="MCListbox (strict)"("ActiveCell"=w314, "CellBG"=w313, "ActiveCell"=w312, "CellBG"=w311) -> ()  [unwired: 2 in, 2 out]
            n158 = call <vilib>:"WPI_DashboardUpdate RPC Info.vi"("Operation"=w307) -> ("update"=w305:bool, "commands"=w304:string[][])  [unwired: 9 in]
            n159 = property on="Command Selection" class="MCListbox (strict)"("ItemNames"=w304) -> ()  [unwired: 2 in, 2 out]
            n160 = property on="Command Params" class="Tbl (strict)"("Active Cell"=w314, "Cell BG Color"=w313, "Active Cell"=w312, "Cell BG Color"=w311) -> ()  [unwired: 2 in, 2 out]
            n161 = call <vilib>:"WPI_DashboardUpdate Command Params.vi"("Update"=w305, "NewVal"=w306, "Commands"=w304, "Param Tbl"=w303) -> ()  [unwired: 7 in, 1 out]
          }
        }
        n162 = case shown="\"\"" w290 {
          tunnel: "/TestMode/TestProgress" ("Name") -> [w317 _]
          tunnel: "/TestMode/TestProgressText" ("Name") -> [w316 _]
          frame Default {
            n163 = call <vilib>:"NT Read Number.vi"("Name"=w317) -> ("Numeric"=w318:dbl)  [unwired: 9 in, 1 out]
            n164 = call <vilib>:"NT Read String.vi"("Name"=w316) -> ("String"=w319:string)  [unwired: 9 in, 1 out]
            n165 = Bundle("Numeric"=w318, "String"=w319) -> (→"Progress":cluster{"Numeric":dbl, "String":string})  [unwired: 1 in]
          }
          frame "" {
            n166 = property on="Progress" class="Clust (strict)"("Visible"=FALSE) -> ()  [unwired: 2 in, 2 out]
            n167 = local write "Test Name"(u16 0) -> ()
          }
        }
        n168 = call <vilib>:"Connextion Info.vi"() -> ("Connected"=→"NT Connection":bool)  [unwired: 10 in, 1 out]
      }
      event "Test Tree": Value Change {
        # "Show appropriate\ncontrols"
        n169 = event-data() -> ("CtlRef"=w328:refnum<vi>, "NewVal"=w326:string)  [unwired: 1 in]
        n170 = call <vilib>:"WPI_UtilitiesGetTreeIOName.vi"("NewVal"=w326, "TreeControl in"=w328) -> ("I/O Name"=w329:string)  [unwired: 9 in]
        n171 = case shown="\"Analog Out\", \"Motor\", \"PWM\"" w329 {
          selector: w329 -> [_ w336 _ w358 w367 _]
          tunnel: w326 -> [_ _ w355 w357 _ w374]
          tunnel: w325 -> [_ _ _ _ _ w373]
          frame Default {
            w331 = FALSE ("Visible")
            w330 = FALSE ("Visible")
            n172 = property on="Motor" class="Clust (strict)"("Visible"=w330) -> ()  [unwired: 2 in, 2 out]
            n173 = property on="Test Ring" class="Ring (strict)"("Visible"=w330) -> ()  [unwired: 2 in, 2 out]
            n174 = property on="Rev/Fwd" class="Clust (strict)"("Visible"=w331) -> ()  [unwired: 2 in, 2 out]
            n175 = property on="On/Off" class="Bool (strict)"("Visible"=w331) -> ()  [unwired: 2 in, 2 out]
            n176 = property on="Test Slider" class="Slide (strict)"("Visible"=w331) -> ()  [unwired: 2 in, 2 out]
          }
          frame "Analog Out", "Motor", "PWM" {
            w337 = FALSE ("Visible")
            n177 = case shown="\"Analog Out\"" w336 {
              tunnel: [1.0 ("Value") -1.0 ("Value") 0.0 ("Value")] -> w335
              tunnel: [255.0 ("Value") 1.0 ("Value") 5.0 ("Value")] -> w334
              tunnel: [128.0 ("Value") 0.0 ("Value") 0.0 ("Value")] -> w333
              tunnel: [64.0 ("Value") 0.5 ("Value") 1.0 ("Value")] -> w332
              frame "PWM" {
              }
              frame "Motor", Default {
              }
              frame "Analog Out" {
              }
            }
            n178 = property on="Motor" class="Clust (strict)"("Visible"=TRUE) -> ()  [unwired: 2 in, 2 out]
            n179 = property on="Value" class="Slide (strict)"("Value"=w333, "Scale.Minimum"=w335, "Scale.Maximum"=w334, "Scale.Increment"=w332) -> ()  [unwired: 2 in, 2 out]
            n180 = property on="On/Off" class="Bool (strict)"("Visible"=w337) -> ()  [unwired: 2 in, 2 out]
            n181 = property on="Test Slider" class="Slide (strict)"("Visible"=w337) -> ()  [unwired: 2 in, 2 out]
            n182 = property on="Test Ring" class="Ring (strict)"("Visible"=w337) -> ()  [unwired: 2 in, 2 out]
            n183 = property on="Rev/Fwd" class="Clust (strict)"("Visible"=w337) -> ()  [unwired: 2 in, 2 out]
          }
          frame "Servo" {
            w353 = FALSE ("Visible")
            n184 = call <vilib>:"NT Read Number.vi"("Name"=w355) -> ("Numeric"=w354:dbl)  [unwired: 9 in, 1 out]
            n185 = property on="Test Slider" class="Slide (strict)"("Visible"=TRUE, "Scale.Maximum"=170.0 ("Scale.Range:Maximum")) -> ()  [unwired: 2 in, 2 out]
            n186 = local write "Test Slider"(w354) -> ()
            n187 = property on="Motor" class="Clust (strict)"("Visible"=w353) -> ()  [unwired: 2 in, 2 out]
            n188 = property on="Rev/Fwd" class="Clust (strict)"("Visible"=w353) -> ()  [unwired: 2 in, 2 out]
            n189 = property on="On/Off" class="Bool (strict)"("Visible"=w353) -> ()  [unwired: 2 in, 2 out]
            n190 = property on="Test Ring" class="Ring (strict)"("Visible"=w353) -> ()  [unwired: 2 in, 2 out]
          }
          frame "Relay", "Solenoid" {
            w356 = FALSE ("Visible")
            n191 = property on="Motor" class="Clust (strict)"("Visible"=w356) -> ()  [unwired: 2 in, 2 out]
            n192 = property on="Test Slider" class="Slide (strict)"("Visible"=w356) -> ()  [unwired: 2 in, 2 out]
            n193 = Search and Replace String(input string=w357, search string="/Value  **", replace string="/Direction") -> (result string=w363:string)  [unwired: 5 in, 3 out]
            n194 = property on="Test Ring" class="Ring (strict)"("Visible"=w356) -> ()  [unwired: 2 in, 2 out]
            n195 = call <vilib>:"NT Read String.vi"("Name"=w363) -> ("String"=w361:string)  [unwired: 9 in, 1 out]
            n196 = Equal?(x="Both directions", y=w361) -> (x = y?=w359:bool)
            n197 = Not(x=w359) -> (.not. x?=w360:bool)
            n198 = property on="Rev/Fwd" class="Clust (strict)"("Visible"=w359) -> ()  [unwired: 2 in, 2 out]
            n199 = property on="On/Off" class="Bool (strict)"("Visible"=w360, "Caption.Text"=w358) -> ()  [unwired: 2 in, 2 out]
          }
          frame "Compressor", "Digital Out" {
            w366 = FALSE ("Visible")
            # "Get direction and finish"
            n200 = property on="Motor" class="Clust (strict)"("Visible"=w366) -> ()  [unwired: 2 in, 2 out]
            n201 = property on="Test Slider" class="Slide (strict)"("Visible"=w366) -> ()  [unwired: 2 in, 2 out]
            n202 = property on="Test Ring" class="Ring (strict)"("Visible"=w366) -> ()  [unwired: 2 in, 2 out]
            n203 = property on="On/Off" class="Bool (strict)"("Visible"=TRUE, "Caption.Text"=w367) -> ()  [unwired: 2 in, 2 out]
            n204 = property on="Rev/Fwd" class="Clust (strict)"("Visible"=FALSE) -> ()  [unwired: 2 in, 2 out]
          }
          frame "Camera" {
            n205 = call <vilib>:"Get Last Path Segment.vi"("String in"=w374) -> ("String out"=w375:string)  [unwired: 10 in]
            n206 = property on="On/Off" class="Bool (strict)"("Visible"=FALSE) -> ()  [unwired: 2 in, 2 out]
            n207 = property on="Motor" class="Clust (strict)"("Visible"=FALSE) -> ()  [unwired: 2 in, 2 out]
            n208 = property on="Rev/Fwd" class="Clust (strict)"("Visible"=FALSE) -> ()  [unwired: 2 in, 2 out]
            n209 = case shown="\"White Balance  **\"" w375 {
              tunnel: w374 -> [w381 w390 w399 w408 w417 _ w423]
              tunnel: w373 -> [w379 w387 w396 w405 w414 _ _]
              frame "Size  **" {
                n210 = Index Array(array=w379) -> (element=w378:cluster{string[]})  [unwired: 1 in]
                n211 = call <vilib>:"NT Read String.vi"("Name"=w381) -> ("String"=w380:string)  [unwired: 9 in, 1 out]
                n212 = Unbundle(w378) -> (w376:string[])
                n213 = Match First String(2:w376, 3:w380) -> (0:w377:i32)  [unwired: 1 out]
                n214 = property on="Test Ring" class="Ring (strict)"("Value"=w377, "Strings []"=w376) -> ()  [unwired: 2 in, 2 out]
                n215 = property on="Test Ring" class="Ring (strict)"("Visible"=TRUE) -> ()  [unwired: 2 in, 2 out]
                n216 = property on="Test Slider" class="Slide (strict)"("Visible"=FALSE) -> ()  [unwired: 2 in, 2 out]
              }
              frame "White Balance  **" {
                n217 = Index Array(array=w387, index=1) -> (element=w388:cluster{string[]})
                n218 = call <vilib>:"NT Read String.vi"("Name"=w390) -> ("String"=w389:string)  [unwired: 9 in, 1 out]
                n219 = Unbundle(w388) -> (w385:string[])
                n220 = Match First String(2:w385, 3:w389) -> (0:w384:i32)  [unwired: 1 out]
                n221 = property on="Test Ring" class="Ring (strict)"("Value"=w384, "Strings []"=w385) -> ()  [unwired: 2 in, 2 out]
                n222 = property on="Test Ring" class="Ring (strict)"("Visible"=TRUE) -> ()  [unwired: 2 in, 2 out]
                n223 = property on="Test Slider" class="Slide (strict)"("Visible"=FALSE) -> ()  [unwired: 2 in, 2 out]
              }
              frame "Exposure  **" {
                n224 = Index Array(array=w396, index=2) -> (element=w397:cluster{string[]})
                n225 = call <vilib>:"NT Read String.vi"("Name"=w399) -> ("String"=w398:string)  [unwired: 9 in, 1 out]
                n226 = Unbundle(w397) -> (w393:string[])
                n227 = Match First String(2:w393, 3:w398) -> (0:w394:i32)  [unwired: 1 out]
                n228 = property on="Test Ring" class="Ring (strict)"("Value"=w394, "Strings []"=w393) -> ()  [unwired: 2 in, 2 out]
                n229 = property on="Test Ring" class="Ring (strict)"("Visible"=TRUE) -> ()  [unwired: 2 in, 2 out]
                n230 = property on="Test Slider" class="Slide (strict)"("Visible"=FALSE) -> ()  [unwired: 2 in, 2 out]
              }
              frame "Exposure Priority  **" {
                n231 = Index Array(array=w405, index=3) -> (element=w406:cluster{string[]})
                n232 = call <vilib>:"NT Read String.vi"("Name"=w408) -> ("String"=w407:string)  [unwired: 9 in, 1 out]
                n233 = Unbundle(w406) -> (w402:string[])
                n234 = Match First String(2:w402, 3:w407) -> (0:w403:i32)  [unwired: 1 out]
                n235 = property on="Test Ring" class="Ring (strict)"("Value"=w403, "Strings []"=w402) -> ()  [unwired: 2 in, 2 out]
                n236 = property on="Test Ring" class="Ring (strict)"("Visible"=TRUE) -> ()  [unwired: 2 in, 2 out]
                n237 = property on="Test Slider" class="Slide (strict)"("Visible"=FALSE) -> ()  [unwired: 2 in, 2 out]
              }
              frame "Color Enable  **" {
                n238 = Index Array(array=w414, index=4) -> (element=w415:cluster{string[]})
                n239 = call <vilib>:"NT Read String.vi"("Name"=w417) -> ("String"=w416:string)  [unwired: 9 in, 1 out]
                n240 = Unbundle(w415) -> (w411:string[])
                n241 = Match First String(2:w411, 3:w416) -> (0:w412:i32)  [unwired: 1 out]
                n242 = property on="Test Ring" class="Ring (strict)"("Value"=w412, "Strings []"=w411) -> ()  [unwired: 2 in, 2 out]
                n243 = property on="Test Ring" class="Ring (strict)"("Visible"=TRUE) -> ()  [unwired: 2 in, 2 out]
                n244 = property on="Test Slider" class="Slide (strict)"("Visible"=FALSE) -> ()  [unwired: 2 in, 2 out]
              }
              frame Default {
                n245 = property on="Test Ring" class="Ring (strict)"("Visible"=FALSE) -> ()  [unwired: 2 in, 2 out]
                n246 = property on="Test Slider" class="Slide (strict)"("Visible"=FALSE) -> ()  [unwired: 2 in, 2 out]
              }
              frame "Brightness  **", "Color Level  **", "Compression  **", "FPS  **", "Sharpness  **" {
                n247 = call <vilib>:"NT Read Number.vi"("Name"=w423) -> ("Numeric"=w422:dbl)  [unwired: 9 in, 1 out]
                n248 = local write "Test Slider"(w422) -> ()
                n249 = property on="Test Slider" class="Slide (strict)"("Visible"=TRUE, "Scale.Maximum"=100.0 ("Scale.Range:Maximum")) -> ()  [unwired: 2 in, 2 out]
                n250 = property on="Test Ring" class="Ring (strict)"("Visible"=FALSE) -> ()  [unwired: 2 in, 2 out]
              }
            }
          }
        }
        n251 = property on="Progress" class="Clust (strict)"("Visible"=FALSE) -> ()  [unwired: 2 in, 2 out]
      }
      event "Test Name": Mouse Enter {
        # "Populate the ring with the list of tests"
        n252 = event-data() -> ()  [unwired: 1 in, 1 out]
        n253 = call <vilib>:"NT Read String Array.vi"("Name"="/TestMode/TestList") -> ("String Array"=w432:string[])  [unwired: 9 in, 1 out]
        n254 = Build Array (concatenate)("Select the test to run...", w432) -> (w431:string[])
        n255 = property on="Test Name" class="Ring (strict)"("Strings []"=w431) -> ()  [unwired: 2 in, 2 out]
      }
      event "Test Name": Value Change {
        w435 = FALSE ("Visible")
        # "Tell the robot the test name to run"
        n256 = event-data() -> ("NewVal"=w439:u16)  [unwired: 1 in]
        n257 = property on="Test Name" class="Ring (strict)"() -> ("Strings []"=w440:string[])  [unwired: 2 in, 2 out]
        n258 = local write "Progress"(T10 {"Test Progress"=0, "Test Progress Text"=""} ("Progress")) -> ()
        n259 = Index Array(array=w440, index=w439) -> (element=w438:string)
        n260 = call <vilib>:"NT Write String.vi"("String"=w438, "Name"="/TestMode/TestName") -> ()  [unwired: 9 in, 1 out]
        n261 = property on="Progress" class="Clust (strict)"("Visible"=TRUE) -> ()  [unwired: 2 in, 2 out]
        n262 = property on="Motor" class="Clust (strict)"("Visible"=w435) -> ()  [unwired: 2 in, 2 out]
        n263 = property on="Test Slider" class="Slide (strict)"("Visible"=w435) -> ()  [unwired: 2 in, 2 out]
        n264 = property on="On/Off" class="Bool (strict)"("Visible"=w435) -> ()  [unwired: 2 in, 2 out]
        n265 = property on="Rev/Fwd" class="Clust (strict)"("Visible"=w435) -> ()  [unwired: 2 in, 2 out]
        n266 = property on="Test Ring" class="Ring (strict)"("Visible"=w435) -> ()  [unwired: 2 in, 2 out]
      }
      event "Select Auto": Mouse Enter {
        # "Populate the combo box with the list of autonomous options"
        n267 = event-data() -> ()  [unwired: 1 in, 1 out]
        n268 = call <vilib>:"NT Read String Array.vi"("Name"="Auto List") -> ("String Array"=w442:string[])  [unwired: 9 in, 1 out]
        n269 = property on="Select Auto" class="CmbBox"("Strings[]"=w442) -> ()  [unwired: 2 in, 2 out]
      }
      event "Select Auto": Value Change {
        # "User modified the Auto Selection. Write to NT variable so robot knows."
        n270 = event-data() -> ("NewVal"=w446:string)  [unwired: 1 in]
        n271 = call <vilib>:"NT Write String.vi"("String"=w446, "Name"="Auto Selector") -> ()  [unwired: 9 in, 1 out]
      }
      event "Command Selection": Value Change {
        # "Get the params and show in table"
        n272 = event-data() -> ("NewVal"=w453:i32)  [unwired: 1 in]
        n273 = property on="Command Selection" class="MCListbox (strict)"() -> ("ItemNames"=w451:string[][])  [unwired: 2 in, 2 out]
        n274 = call <vilib>:"WPI_DashboardUpdate Command Params.vi"("NewVal"=w453, "Commands"=w451, "Param Tbl"=w452) -> ()  [unwired: 8 in, 1 out]
      }
      event "Execute Command": Value Change {
        # "Started one, Unique ID holds\nresponse"
        n275 = event-data() -> ()  [unwired: 1 in, 1 out]
        n276 = property on="Command Selection" class="MCListbox (strict)"() -> ("ItemNames"=w465:string[][])  [unwired: 2 in, 2 out]
        n277 = Index Array(array=w465, index (row)="Command Selection", index (col)=0) -> (element=w463:string)
        n278 = call <vilib>:"Invoke Commands.vi"("Command Params"="Command Params", "Function Name"=w463) -> ("Params"=w459:u8, "Started"=w458:bool)  [unwired: 7 in, 1 out]
        n279 = Array Subset(array="Command Params", length (row)=w459) -> (w460:string[][])  [unwired: 3 in]
        n280 = Select(t="Executing" ("Cmd Status"), s=w458, f="" ("Cmd Status")) -> (s? t:f=→"Cmd Status":string)
      }
      event "Command Selection": Double Click {
        n281 = event-data() -> ("Row"=w475:i32)  [unwired: 1 in]
        n282 = property on="Command Selection" class="MCListbox (strict)"() -> ("ItemNames"=w478:string[][])  [unwired: 2 in, 2 out]
        n283 = local read "Command Params"() -> (w473:string[][])
        n284 = Index Array(array=w478, index (row)=w475, index (col)=0) -> (element=w476:string)
        n285 = call <vilib>:"Invoke Commands.vi"("Command Params"=w473, "Function Name"=w476) -> ("Params"=w472:u8, "Started"=w467:bool)  [unwired: 7 in, 1 out]
        n286 = Array Subset(array=w473, length (row)=w472) -> (w471:string[][])  [unwired: 3 in]
        n287 = Select(t="Executing" ("Cmd Status"), s=w467, f="" ("Cmd Status")) -> (s? t:f=w468:string)
        n288 = local write "Cmd Status"(w468) -> ()
      }
      event "CheckList": Double Click {
        # "Shift clears all"
        # "Update symbols on the listbox"
        n289 = event-data() -> ("PlatMods.Shift"=w481:bool, "Row"=w483:i32)  [unwired: 1 in]
        n290 = case shown="True" w481 {
          tunnel: w483 -> [w487 _]
          tunnel: 1 -> [w486 _]
          frame False {
            n291 = property on="CheckList" class="LstBox (strict)"() -> ("Item Symbols"=w485:i32[])  [unwired: 2 in, 2 out]
            n292 = Replace Array Subset(array=w485, new element=w486, index=w487) -> (w484:i32[])
            n293 = property on="CheckList" class="LstBox (strict)"("Item Symbols"=w484) -> ()  [unwired: 2 in, 2 out]
          }
          frame True {
            w488 = 0 ("Top Row")
            n294 = property on="CheckList" class="LstBox (strict)"() -> ("Number of Rows"=w490:u32)  [unwired: 2 in, 2 out]
            n295 = Initialize Array(0, w490) -> (w489:i32[])
            n296 = property on="CheckList" class="LstBox (strict)"("Top Row"=w488, "Value"=w488, "Item Symbols"=w489) -> ()  [unwired: 2 in, 2 out]
          }
        }
      }
      event "CheckList": Key Down {
        # "Update symbols on the listbox\nLeft and right keys check and uncheck"
        n297 = event-data() -> ("VKey"=w495:T27)  [unwired: 1 in]
        n298 = case shown="\"Left\", \"Right\"" w495 {
          selector: w495 -> [w500 _]
          tunnel: eventvkey."Left" ("VKey") -> [w498 _]
          frame "Left", "Right" {
            n299 = Equal?(x=w498, y=w500) -> (x = y?=w499:bool)
            n300 = Select(t=0, s=w499, f=1) -> (s? t:f=w501:i32)
            n301 = property on="CheckList" class="LstBox (strict)"() -> ("Item Symbols"=w504:i32[])  [unwired: 2 in, 2 out]
            n302 = Replace Array Subset(array=w504, new element=w501, index="CheckList") -> (w503:i32[])
            n303 = property on="CheckList" class="LstBox (strict)"("Item Symbols"=w503) -> ()  [unwired: 2 in, 2 out]
          }
          frame Default {
          }
        }
      }
      event "DB Camera Config": Value Change {
        # "Show or hide the cluster of controls, store in ini file"
        n304 = event-data() -> ("NewVal"=w509:bool)  [unwired: 1 in]
        n305 = case shown="False" w509 {
          tunnel: w508 -> [w518 _]
          tunnel: [w511 w529] -> w507
          tunnel: w506 -> [w510 w529]
          frame False {
            w525 = "Camera"
            w528 = FALSE ("Visible")
            n306 = local read "Camera Settings"() -> (w517:T2)
            n307 = Index Array(array=w518) -> (element=w521:cluster{string[]})  [unwired: 1 in]
            n308 = Unbundle(w517) -> ("Frame Rate"=w516:i32, "Compression"=w515:i32, "Size"=w519:u16)
            n309 = Unbundle(w521) -> (w520:string[])
            n310 = Index Array(array=w520, index=w519) -> (element=w514:string)
            n311 = call-poly <vilib>:"Write Key.vi"("section"=w525, "value"=w514, "key"="Size", "refnum"=w510) -> ("refnum out"=w527:T21)  [unwired: 2 in, 5 out]
            n312 = call-poly <vilib>:"Write Key.vi"("section"=w525, "value"=w516, "key"="FrameRate", "refnum"=w527) -> ("refnum out"=w526:T21)  [unwired: 1 in, 6 out]
            n313 = property on="Camera Settings" class="Clust (strict)"("Visible"=w528) -> ()  [unwired: 2 in, 2 out]
            n314 = local write "DB Camera Config"(w528) -> ()
            n315 = call-poly <vilib>:"Write Key.vi"("section"=w525, "value"=w515, "key"="Compression", "refnum"=w526) -> ("refnum out"=w512:T21)  [unwired: 1 in, 6 out]
            n316 = call <vilib>:"Close Config Data.vi"("refnum"=w512) -> ("file path"=w513:path)  [unwired: 2 in, 8 out]
            n317 = call <vilib>:"Open Config Data.vi"("configuration file path"=w513) -> ("refnum"=w511:T21)  [unwired: 8 in, 2 out]
          }
          frame True {
            n318 = property on="Camera Settings" class="Clust (strict)"("Visible"=TRUE) -> ()  [unwired: 2 in, 2 out]
          }
        }
      }
      event "Camera Settings": Value Change {
        # "Update summary string when any elements of DB camera change"
        n319 = event-data() -> ("NewVal"=w543:T2)  [unwired: 1 in]
        n320 = Index Array(array=w539) -> (element=w538:cluster{string[]})  [unwired: 1 in]
        n321 = Unbundle(w543) -> ("Frame Rate"=w534:i32, "Compression"=w533:i32, "Size"=w536:u16)
        n322 = Unbundle(w538) -> (w537:string[])
        n323 = Index Array(array=w537, index=w536) -> (element=w535:string)
        n324 = Format Into String(format string="%s   %dfps   %d%%", w535, w534, w533) -> (resulting string=w540:string)  [unwired: 2 in, 1 out]
        n325 = Build Array(w540) -> (w541:string[])
        n326 = property on="DB Camera Config" class="Bool (strict)"("Strings [4]"=w541) -> ()  [unwired: 2 in, 2 out]
      }
      event "Motor.Enable": Value Change {
        # "When the test mode otor enable helper is set, update that\ntree row item's value"
        n327 = event-data() -> ("NewVal"=w550:bool)  [unwired: 1 in]
        n328 = Unbundle("Motor") -> ("Value"=w549:dbl)  [unwired: 1 out]
        n329 = Select(t=w549, s=w550, f=0.0) -> (s? t:f=w547:dbl)
        n330 = call <vilib>:"NT Write Number.vi"("Numeric"=w547, "Name"=w546) -> ()  [unwired: 9 in, 1 out]
      }
      event "Test Slider": Value Change {
        # "When the test mode slider helper is set, update that\ntree row item's value"
        n331 = event-data() -> ("NewVal"=w554:dbl)  [unwired: 1 in]
        n332 = call <vilib>:"NT Write Number.vi"("Numeric"=w554, "Name"=w555) -> ()  [unwired: 9 in, 1 out]
      }
      event "On/Off": Value Change {
        # "When the test mode on/off helper value is set, update that\ntree row item's value"
        n333 = event-data() -> ("NewVal"=w560:bool)  [unwired: 1 in]
        n334 = Boolean To (0,1)(Boolean=w560) -> (0, 1=w559:i16)
        n335 = call <vilib>:"NT Write Number.vi"("Numeric"=w559, "Name"=w558) -> ()  [unwired: 9 in, 1 out]
      }
      event "Rev/Fwd": Value Change {
        # "When the test mode helper value for relays is set, update that\ntree row item's value"
        n336 = event-data() -> ("NewVal.Forward"=w569:bool, "NewVal.Reverse"=w568:bool)  [unwired: 1 in]
        n337 = Boolean To (0,1)(Boolean=w569) -> (0, 1=w565:i16)
        n338 = Boolean To (0,1)(Boolean=w568) -> (0, 1=w567:i16)
        n339 = Negate(x=w567) -> (-x=w566:i16)
        n340 = Add(x=w565, y=w566) -> (x+y=w564:i16)
        n341 = call <vilib>:"NT Write Number.vi"("Numeric"=w564, "Name"=w563) -> ()  [unwired: 9 in, 1 out]
      }
      event "Test Ring": Value Change {
        # "When a test mode helper value is selected from the ring,\nset the tree item's variable to the string value"
        n342 = event-data() -> ("NewVal"=w574:u16)  [unwired: 1 in]
        n343 = property on="Test Ring" class="Ring (strict)"() -> ("Strings []"=w575:string[])  [unwired: 2 in, 2 out]
        n344 = Index Array(array=w575, index=w574) -> (element=w573:string)
        n345 = call <vilib>:"NT Write String.vi"("String"=w573, "Name"=w572) -> ()  [unwired: 9 in, 1 out]
      }
      event "Rec Mode": Value Change {
        # "Update globals for recording mode and path to read log from.\nClear when logging and let NetworkTables set path for vision to\nuse."
        n346 = event-data() -> ("NewVal"=w587:enum32{"Stop", "Record", "Playback"})  [unwired: 1 in]
        n347 = global write "WPI_DashboardLogging Global.vi" "Logging Filename"(path "") -> ()
        n348 = global write "WPI_DashboardLogging Global.vi" "Recording"(w587) -> ()
        n349 = case shown="\"Playback\"" w587 {
          tunnel: w586 -> [_ w589 w598]
          tunnel: [_ _ w597] -> w583
          tunnel: [_ _ w596] -> _
          tunnel: w581 -> [_ _ w594]
          tunnel: cluster{i32, i32} {-250, 170} -> [_ _ w593]
          tunnel: [_ _ T28 {"Image Size"=TRUE, "Image Type"=TRUE, "Pixel Value"=TRUE, "ROI Information"=TRUE, "Zoom Factor"=FALSE} ("Image Information Shown:All Elements")] -> w579
          tunnel: [_ _ TRUE ("Zoom Factor")] -> w578
          tunnel: w577 -> [_ _ w590]
          frame Default {
          }
          frame "Stop", "Record" {
            # "Place Window too"
            n350 = invoke class="VI" method="FP.Close"(reference=w589) -> (reference out=w588:refnum<vi>)  [unwired: 2 in, 2 out]
            n351 = invoke class="VI" method="Abort VI"(reference=w588) -> ()  [unwired: 2 in, 3 out]
          }
          frame "Playback" {
            n352 = call "Open Playback Panel.vi"("Offset"=w593, "DB VI Ref"=w594, "Playback in"=w598) -> ("Playback out"=w595:refnum<vi>)  [unwired: 8 in]
            n353 = register-events(w595, w590) -> (reference out=w597:refnum<event-registration>, error out=w596:errorcluster)  [unwired: 2 in]
          }
        }
        n354 = property on="Camera Image" class="ImageControl"("Image Information Shown"=w579, "Image Information Visible"=w578) -> ()  [unwired: 2 in, 2 out]
        n355 = call <vilib>:"WPI_DashboardNT Log FieldName Cache.vi"("Operation"=enum16{"Lookup/Add", "Index", "Clear"}."Clear") -> ()  [unwired: 8 in, 3 out]
      }
      event Panel Close {
        w600 = enum32{"Stop", "Record", "Playback"}."Stop" ("Rec Mode")
        # "Playback window has been closed, abort"
        n356 = event-data() -> ()  [unwired: 1 in, 4 out]
        n357 = local write "Rec Mode"(w600) -> ()
        n358 = global write "WPI_DashboardLogging Global.vi" "Recording"(w600) -> ()
      }
      event Panel Close {
        # "Abort playback window and ourself"
        n359 = event-data() -> ()  [unwired: 1 in, 4 out]
        n360 = invoke class="VI" method="FP.Close"(reference=w606) -> (reference out=w605:refnum<vi>)  [unwired: 2 in, 2 out]
        n361 = invoke class="VI" method="Abort VI"(reference=w605) -> (error out=w604:errorcluster)  [unwired: 2 in, 2 out]
        n362 = invoke class="VI" method="Abort VI"(error in=w604) -> ()  [unwired: 2 in, 3 out]
      }
      event User Event {
        n363 = event-data() -> ("IDs"=w614:cluster{"RPC field ID":u16, "Unique ID":u16}, "String"=w613:string)  [unwired: 1 in]
        n364 = Bundle("IDs"=w614, "String"=w613) -> (w612:T12)  [unwired: 1 in]
        n365 = call <vilib>:"Retrieve RPC Response.vi"("RPC Response"=w612) -> ("Output"=w609:string[][])  [unwired: 10 in]
        n366 = Build Array (concatenate)(w607, w609) -> (w608:string[][])
        n367 = local write "Command Params"(w608) -> ()
        n368 = local write "Cmd Status"("" ("Cmd Status")) -> ()
      }
      event "Vision": Value Change {
        # "Enable/Disable Compression slider.\nHW USB is hard-coded into the camera"
        n369 = event-data() -> ("NewVal"=w621:u16)  [unwired: 1 in]
        n370 = Equal?(x=w621, y=u32 2 ("milliseconds to wait")) -> (x = y?=w619:bool)
        n371 = Select(t=T29."Disabled and Grayed Out" ("Disabled"), s=w619, f=T29."Enabled" ("Disabled")) -> (s? t:f=w616:T29)
        n372 = property on="Compression" class="Slide (strict)"("DisabledEnum"=w616) -> ()  [unwired: 2 in, 2 out]
      }
      event "Tree": Double Click {
        n373 = event-data() -> ("PlatMods"=w626:T32, "Tag"=w625:string)  [unwired: 1 in]
        n374 = Unbundle(w626) -> ("Shift"=w624:bool)  [unwired: 4 out]
        n375 = Not(x=w624) -> (.not. x?=w623:bool)
        n376 = call <vilib>:"NT Update Persistence.vi"("Persistence"=w623, "Name"=w625) -> ()  [unwired: 9 in, 1 out]
      }
    }
  }
  n377 = while {
    tunnel: w66 -> [w630]
    i -> [w633]
    stop <- FALSE stop-if-true
    n378 = Wait (ms)(milliseconds to wait=u32 100) -> ()  [unwired: 1 out]
    n379 = case shown="\"Playback\"" "Rec Mode" {
      tunnel: w633 -> [_ _ w648]
      tunnel: [u32 2829099 ("Base Color") u32 11141120 ("Target Color") w637] -> w629
      frame "Stop", Default {
        # "Reset the color, extra updates don't cost much"
      }
      frame "Record" {
      }
      frame "Playback" {
        # "Playback"
        n380 = Quotient & Remainder(x=w648, y=u32 50 ("milliseconds to wait")) -> (x-y*floor(x/y)=w644:u32)  [unwired: 1 out]
        n381 = Divide(x=w644, y=u32 50 ("milliseconds to wait")) -> (x/y=w641:dbl)
        n382 = Multiply(x=6.283185307179586, y=w641) -> (x*y=w646:dbl)
        n383 = Sine(x=w646) -> (sin(x)=w645:dbl)
        n384 = Absolute Value(x=w645) -> (abs(x)=w638:dbl)
        n385 = call "Interpolate RGB Color.vi"("Proportion"=w638, "Target Color"=u32 30976, "Base Color"=u32 2829099) -> ("Result Color"=w637:u32)  [unwired: 8 in]
      }
    }
    n386 = property class="Pane"(reference=w630, "PaneColor"=w629) -> ()  [unwired: 1 in, 2 out]
  }
  n387 = property on="On/Off" class="Bool (strict)"("Visible"=w34) -> ()  [unwired: 2 in, 2 out]
  n388 = property on="Motor" class="Clust (strict)"("Visible"=w34) -> ()  [unwired: 2 in, 2 out]
  n389 = property on="Progress" class="Clust (strict)"("Visible"=w34) -> ()  [unwired: 2 in, 2 out]
  n390 = property on="Test Ring" class="Ring (strict)"("Visible"=w34) -> ()  [unwired: 2 in, 2 out]
  n391 = property on="Rev/Fwd" class="Clust (strict)"("Visible"=w34) -> ()  [unwired: 2 in, 2 out]
  n392 = property on="Camera Settings" class="Clust (strict)"("Visible"=w34) -> ()  [unwired: 2 in, 2 out]
  n393 = local write "DB Camera Config"(w34) -> ()
  n394 = local write "Command Params"(string[][] [] ("Command Params")) -> ()
  n395 = global write "WPI_DashboardLogging Global.vi" "Recording"(w60) -> ()
  n396 = local write "Rec Mode"(w60) -> ()
  n397 = while {
    tunnel: u16 1741 ("timeout ms (25000)") -> [w650]
    stop <- FALSE stop-if-true
    n398 = TCP Create Listener(10:w650) -> (0:w649:errorcluster, 3:w651:refnum<k5>)  [unwired: 4 in, 1 out]
    n399 = case shown="No Error" w649 {
      selector: w649 -> [w653 _]
      tunnel: w651 -> [w654 _]
      frame No Error {
        n400 = while {
          tunnel: w654 -> [w657]
          tunnel: w653 -> [w656]
          stop <- FALSE stop-if-true
          n401 = TCP Wait On Listener(8:w656, 11:w657) -> (0:w658:errorcluster, 4:w659:refnum<k5>)  [unwired: 2 in, 3 out]
          n402 = local write "TCP"(w659) -> ()
          n403 = case shown="No Error" w658 {
            frame No Error {
            }
            frame Error {
              n404 = Wait (ms)(milliseconds to wait=u32 1000) -> ()  [unwired: 1 out]
            }
          }
        }
      }
      frame Error {
        n405 = Wait (ms)(milliseconds to wait=u32 1000) -> ()  [unwired: 1 out]
      }
    }
  }
  n406 = local write "Command Selection"(u16 0 ("milliseconds to wait")) -> ()
